vi "VIE.Module.Queued Message Handler.initialize.QueuedMessageHandler.vi"(8 "error in (no error)":errorcluster, 9 "State Queue Log FilePath (\"\" = Do Not Log)":path, 10 "Initial State Queue (empty)":string[](array[string])) -> (0 "error out":errorcluster, 2 "QueuedMessageHandler.dqGOOPClass (out)":T1)   [LabVIEW 2010, in "VIE.Module.Queued Message Handler.QueuedMessageHandler.dqGOOPClass.lvlib"]
uses:
  VIE.Module.Queued Message Handler.QueuedMessageHandler.dqGOOPClass.lvlib
  VIE.Module.Queued Message Handler.dqClass_ObjectReference.ctl
  VIE.Module.Queued Message Handler.[enqueue].State.PolyChild.QueuedMessageHandler.vi
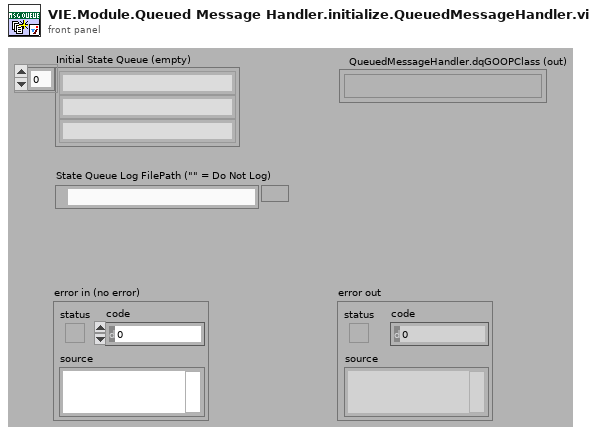
[diagram p1: front panel]
types:
  T1 = typedef "VIE.Module.Queued Message Handler.QueuedMessageHandler.dqGOOPClass.lvlib/VIE.Module.Queued Message Handler.dqClass_ObjectReference.ctl" = refnum<k1>
  T2 = typedef "VIE.Module.Queued Message Handler.QueuedMessageHandler.dqGOOPClass.lvlib/VIE.Module.Queued Message Handler.dqClass_ObjectData.ctl" = cluster{"Message Queue":refnum<queue>, "Log File Refnum":refnum<file>}
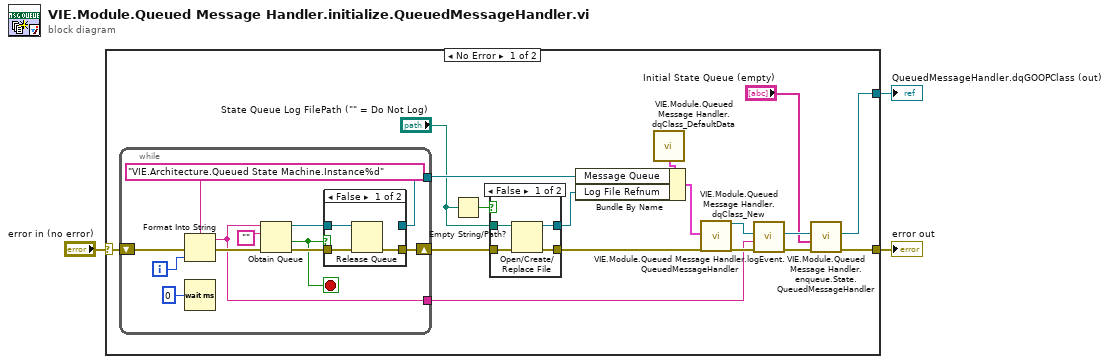
[diagram p0: block diagram]
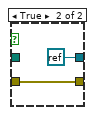
[diagram p2: hidden frame]
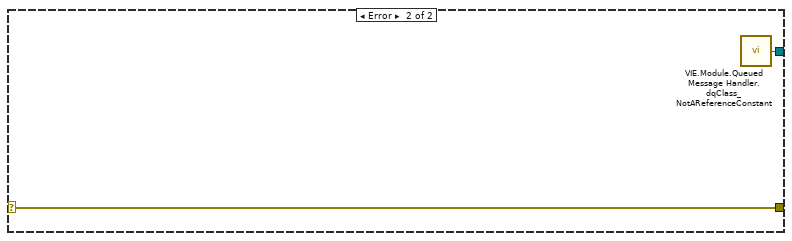
[diagram p4: hidden frame]
diagram:
  n1 = case shown="No Error" "error in (no error)" {
    selector: "error in (no error)" -> [w20 w45]
    tunnel: [w9 w45] -> w2
    tunnel: [w11 w44] -> w1
    frame No Error {
      n2 = while {
        shift-right: [w33] -> w8
        shift-left: w20 -> [w31]
        tunnel: [w30] -> w19
        tunnel: [w27] -> w14
        i -> [w28]
        stop <- w32 stop-if-true
        n3 = Format Into String(format string="VIE.Architecture.Queued State Machine.Instance%d", error in=w31, w28) -> (resulting string=w27:string, error out=w36:errorcluster)  [unwired: 1 in]
        n4 = Wait (ms)(milliseconds to wait=u32 0) -> ()  [unwired: 1 out]
        n5 = Obtain Queue(name (unnamed)=w27, element data type="", error in (no error)=w36) -> (queue out=w34:refnum<queue>, created new?=w32:bool, error out=w35:errorcluster)  [unwired: 2 in]
        n6 = case shown="False" w32 {
          tunnel: w35 -> [w41 w43]
          tunnel: w34 -> [w40 w42]
          tunnel: [w39 w43] -> w33
          tunnel: [_ w42] -> w30
          frame False {
            n7 = Release Queue(queue=w40, error in (no error)=w41) -> (error out=w39:errorcluster)  [unwired: 1 in, 2 out]
          }
          frame True {
          }
        }
      }
      n8 = Empty String/Path?(string/path="State Queue Log FilePath (\"\" = Do Not Log)") -> (empty?=w5:bool)
      n9 = case shown="False" w5 {
        tunnel: w8 -> [w24 w25]
        tunnel: [w23 w25] -> w7
        tunnel: [w22 refnum<k0> refnum] -> w6
        tunnel: "State Queue Log FilePath (\"\" = Do Not Log)" -> [w21 _]
        frame False {
          n10 = Open/Create/Replace File(file path (use dialog)=w21, error in=w24) -> (refnum out=w22:refnum<file>, error out=w23:errorcluster)  [unwired: 4 in, 1 out]
        }
        frame True {
        }
      }
      n11 = call "VIE.Module.Queued Message Handler.dqClass_DefaultData.vi"() -> ("data"=w18:T2)
      n12 = Bundle By Name(cluster=w18, "Message Queue"=w19, "Log File Refnum"=w6) -> (w16:T2)
      n13 = call "VIE.Module.Queued Message Handler.dqClass_New.vi"("data"=w16, "error in (no error)"=w7) -> ("reference"=w15:T1, "error out"=w17:errorcluster)  [unwired: 16 in]
      n14 = call "VIE.Module.Queued Message Handler.logEvent.QueuedMessageHandler.vi"("error in (no error)"=w17, "Event to Log"=w14, "QueuedMessageHandler.dqGOOPClass (in)"=w15) -> ("error out"=w13:errorcluster, "QueuedMessageHandler.dqGOOPClass (out)"=w12:T1)  [unwired: 7 in]
      n15 = call-poly "VIE.Module.Queued Message Handler.enqueue.State.QueuedMessageHandler.vi"("error in (no error)"=w13, "States to Enqueue"="Initial State Queue (empty)", "QueuedMessageHandler.dqGOOPClass (in)"=w12) -> ("error out"=w9:errorcluster, "QueuedMessageHandler.dqGOOPClass (out)"=w11:T1)  [unwired: 7 in]
    }
    frame Error {
      n16 = call "VIE.Module.Queued Message Handler.dqClass_NotAReferenceConstant.vi"() -> ("reference"=w44:T1)
    }
  }
  "error out" <- w2
  "QueuedMessageHandler.dqGOOPClass (out)" <- w1
